vi "Get Display Name for Cfg file.vi"(8 "error in (no error)":errorcluster, 11 "file path":path) -> (0 "error out":errorcluster, 3 "display string":string)   [LabVIEW 2021, in "Audio Popup UI.lvlib"]
uses:
  Audio Popup UI.lvlib
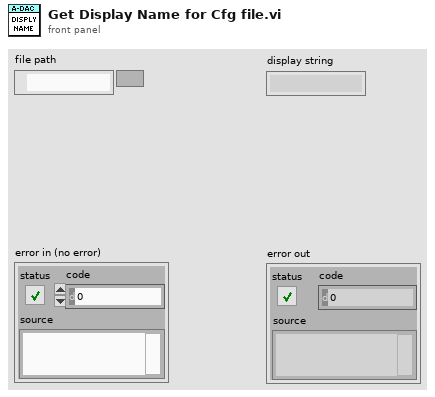
[diagram p1: front panel]
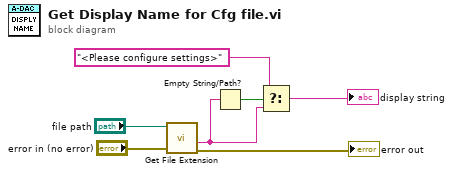
[diagram p0: block diagram]
diagram:
  n1 = call <vilib>:"Get File Extension.vi"("error in (no error)"="error in (no error)", "file"="file path") -> ("error out"=→"error out":errorcluster, "filename without extension"=w4:string)  [unwired: 5 in, 3 out]
  n2 = Empty String/Path?(string/path=w4) -> (empty?=w5:bool)
  n3 = Select(t="<Please configure settings>", s=w5, f=w4) -> (s? t:f=→"display string":string)
